vi "test2_2.vi"() -> ()   [LabVIEW 2010]
doc: "This example shows how to use the instrument's output voltage sweep mode. The actual voltage levels and actual current levels are returned as well as whether over current protection (OCP) has been tripped."
uses:
  <instrlib>/Agilent B2900 Series/Public/Configure/Measurement/Configure Measurement (Current).vi
  <instrlib>/Agilent B2900 Series/Public/Data/Low Level/Fetch Measurement (Multiple Points).vi
  <instrlib>/Agilent B2900 Series/Agilent B2900 Series.lvlib
panel:
  out "Resistance":dbl[](graph)
  out "Resistance":dbl[](array[numeric])
  out "Current vs Voltage":cluster{"Y":dbl[], "Y":dbl[]}[](graph)
  in  "Sweep Range Mode (2: Auto)":i32(ring)=2 items=["Best", "Fix", "Auto"]
  in  "Sweep Number of Steps (7)":i32=7
  in  "Sweep Stop (10 V)":dbl=10.0
  in  "Sweep Start (3 V)":dbl=3.0
  in  "Sweep Output Mode (0: Linear Single)":i32(ring) items=["Linear Single", "Linear Double", "Log Single", "Log Double"]
  out "Actual Voltage Levels (V)":dbl[](array[numeric])
  out "Actual Current Levels (A)":dbl[](array[numeric])
  out "OCP Tripped?":bool
  in  "Current NPLC (0.1)":dbl=0.1
  in  "Trigger Source (0: Auto-Internal)":i32(ring) items=["Auto-Internal", "Bus", "Timer", "INT1", "INT2", "LAN", "EXT1", "EXT2", "EXT3", "EXT4", "EXT5", "EXT6", "EXT7", "EXT8", "EXT9", "EXT10", "EXT11", "EXT12", "EXT13", "EXT14"]
  in  "Enable Output Protection(T: Enable)":bool=TRUE
  in  "Compliance Current (0.0001 A)":dbl=0.0001 format="%_3g"
  in  "Channel (0: Channel 1)":i32(ring) items=["Channel 1", "Channel 2"]
  in  "VISA resource name":refnum<visa-resource-name>
  # "(c) 2011-2013 National Instruments.  ALL RIGHTS RESERVED."
  # "Output Settings"
  # "Compliance Protection"
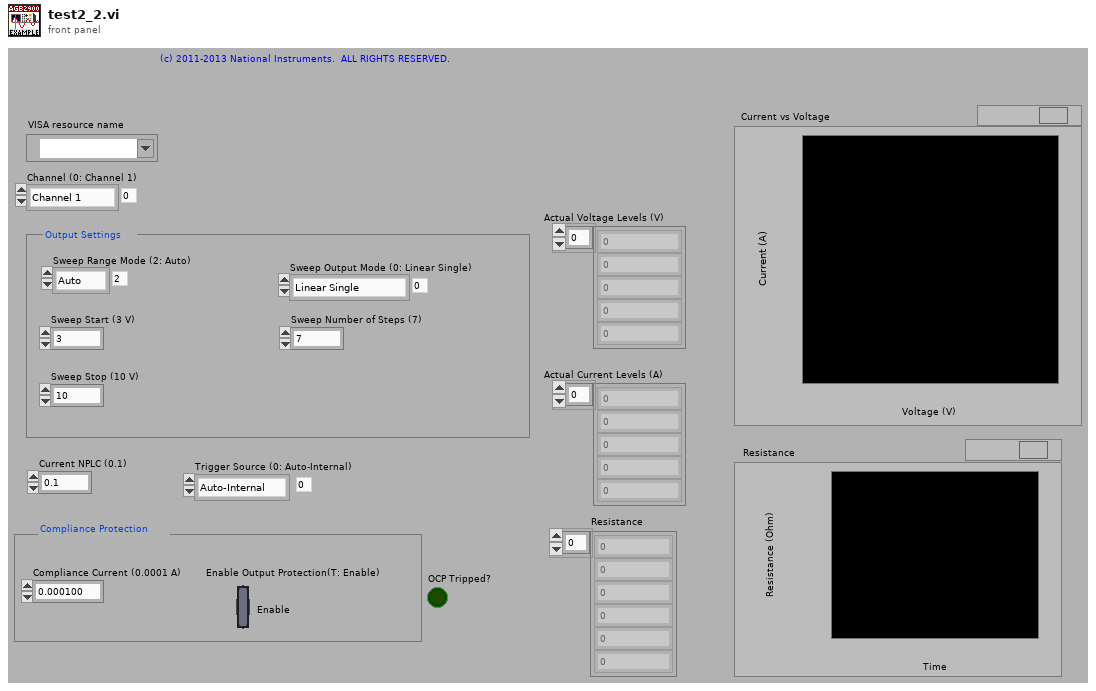
[diagram p1: front panel]
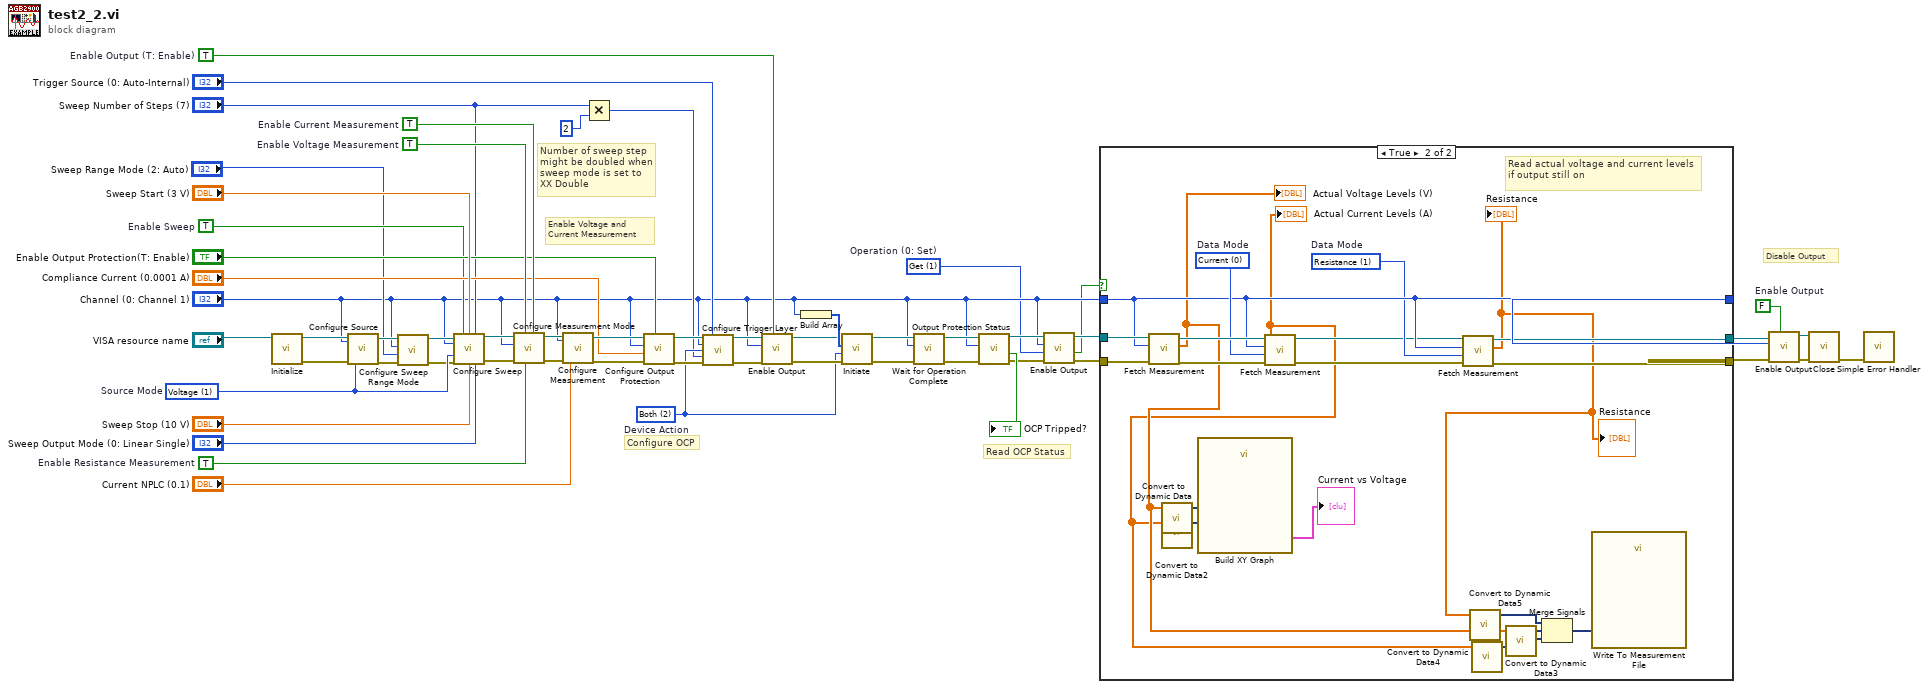
[diagram p0: block diagram]
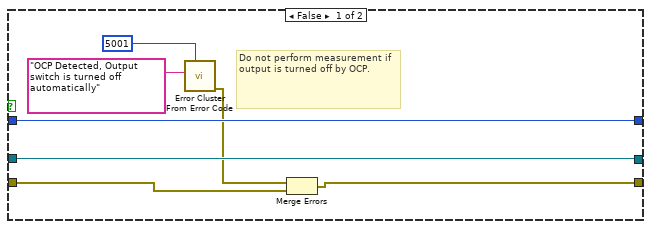
[diagram p2: hidden frame]
diagram:
  w3 = 1 items=["Set", "Get"]  # Operation (0: Set)
  w27 = TRUE  # Enable Current Measurement
  w28 = TRUE  # Enable Voltage Measurement
  w1 = FALSE  # Enable Output
  w26 = 2 items=["Acquire", "Transient", "Both"]  # Device Action
  w31 = TRUE  # Enable Resistance Measurement
  w21 = 1 items=["Current", "Voltage"]  # Source Mode
  w17 = TRUE  # Enable Sweep
  w55 = TRUE  # Enable Output (T: Enable)
  # "Number of sweep step \nmight be doubled when \nsweep mode is set to \nXX Double"
  # "Disable Output"
  # "Read OCP Status"
  # "Enable Voltage and \nCurrent Measurement"
  # "Configure OCP"
  n1 = call <instrlib>:"Initialize.vi"("VISA resource name"="VISA resource name") -> ("error out"=w29:errorcluster, "VISA resource name out"=w30:refnum<visa-resource-name>)  [unwired: 9 in]
  n2 = call <instrlib>:"Configure Source.vi"("VISA resource name"=w30, "Channel (0: Channel 1)"="Channel (0: Channel 1)", "error in (no error)"=w29, "Source Mode (1: Voltage)"=w21) -> ("VISA resource name out"=w15:refnum<visa-resource-name>, "error out"=w12:errorcluster)  [unwired: 14 in]
  n3 = call <instrlib>:"Configure Sweep Range Mode.vi"("error in (no error)"=w12, "Sweep Range Mode (2: Auto)"="Sweep Range Mode (2: Auto)", "Channel (0: Channel 1)"="Channel (0: Channel 1)", "VISA resource name"=w15) -> ("error out"=w13:errorcluster, "VISA resource name out"=w14:refnum<visa-resource-name>)  [unwired: 6 in]
  n4 = call <instrlib>:"Configure Sweep.vi"("VISA resource name"=w14, "Enable Sweep (F: Disable)"=w17, "Sweep Start (0)"="Sweep Start (3 V)", "Sweep Number of Steps (1)"="Sweep Number of Steps (7)", "Channel (0: Channel 1)"="Channel (0: Channel 1)", "Sweep Setting Mode (1: Voltage)"=w21, "error in (no error)"=w13, "Sweep Stop (0)"="Sweep Stop (10 V)", "Sweep Output Mode (0: Linear Single)"="Sweep Output Mode (0: Linear Single)") -> ("VISA resource name out"=w19:refnum<visa-resource-name>, "error out"=w18:errorcluster)  [unwired: 5 in]
  n5 = call <instrlib>:"Configure Measurement Mode.vi"("Enable Current Measurement (T: Enable)"=w27, "Enable Resistance Measurement (F: Disable)"=w31, "Enable Voltage Measurement (T: Enable)"=w28, "error in (no error)"=w18, "Channel (0: Channel 1)"="Channel (0: Channel 1)", "VISA resource name"=w19) -> ("error out"=w51:errorcluster, "VISA resource name out"=w52:refnum<visa-resource-name>)  [unwired: 4 in]
  n6 = call-poly <instrlib>:"Configure Measurement.vi"("VISA resource name"=w52, "Channel (0: Channel 1)"="Channel (0: Channel 1)", "error in (no error)"=w51, "Current NPLC (0.1)"="Current NPLC (0.1)") -> ("VISA resource name out"=w39:refnum<visa-resource-name>, "error out"=w38:errorcluster)  [unwired: 14 in]
  n7 = Multiply(x="Sweep Number of Steps (7)", y=2) -> (x*y=w24:i32)
  n8 = call <instrlib>:"Configure Output Protection.vi"("Enable Output Protection (T: Enable)"="Enable Output Protection(T: Enable)", "error in (no error)"=w38, "Compliance Current (0.0001 A)"="Compliance Current (0.0001 A)", "Channel (0: Channel 1)"="Channel (0: Channel 1)", "VISA resource name"=w39) -> ("error out"=w36:errorcluster, "VISA resource name out"=w37:refnum<visa-resource-name>)  [unwired: 5 in]
  n9 = call <instrlib>:"Configure Trigger Layer.vi"("VISA resource name"=w37, "Trigger Source (0: Auto-Internal)"="Trigger Source (0: Auto-Internal)", "Channel (0: Channel 1)"="Channel (0: Channel 1)", "Device Action (2: Both)"=w26, "Trigger Count (1)"=w24, "error in (no error)"=w36) -> ("VISA resource name out"=w35:refnum<visa-resource-name>, "error out"=w34:errorcluster)  [unwired: 8 in]
  n10 = call <instrlib>:"Enable Output.vi"("Enable Output (T: Enable)"=w55, "error in (no error)"=w34, "Channel (0: Channel 1)"="Channel (0: Channel 1)", "VISA resource name"=w35) -> ("error out"=w53:errorcluster, "VISA resource name out"=w54:refnum<visa-resource-name>)  [unwired: 5 in, 1 out]
  n11 = Build Array("Channel (0: Channel 1)") -> (w56:i32[])
  n12 = call <instrlib>:"Initiate.vi"("error in (no error)"=w53, "Device Action (2: Both)"=w26, "Channel List ({Channel1})"=w56, "VISA resource name"=w54) -> ("error out"=w32:errorcluster, "VISA resource name out"=w33:refnum<visa-resource-name>)  [unwired: 6 in]
  n13 = call <instrlib>:"Wait for Operation Complete.vi"("error in (no error)"=w32, "Channel (0: Channel 1)"="Channel (0: Channel 1)", "VISA resource name"=w33) -> ("error out"=w42:errorcluster, "VISA resource name out"=w43:refnum<visa-resource-name>)  [unwired: 7 in]
  n14 = call <instrlib>:"Output Protection Status.vi"("error in (no error)"=w42, "Channel (0: Channel 1)"="Channel (0: Channel 1)", "VISA resource name"=w43) -> ("error out"=w5:errorcluster, "OCP Tripped?"=→"OCP Tripped?":bool, "VISA resource name out"=w8:refnum<visa-resource-name>)  [unwired: 5 in, 1 out]
  n15 = call <instrlib>:"Enable Output.vi"("error in (no error)"=w5, "Operation (0: Set)"=w3, "Channel (0: Channel 1)"="Channel (0: Channel 1)", "VISA resource name"=w8) -> ("error out"=w7:errorcluster, "Output Enabled?"=w2:bool, "VISA resource name out"=w6:refnum<visa-resource-name>)  [unwired: 5 in]
  n16 = case shown="True" w2 {
    tunnel: w6 -> [w63 w85]
    tunnel: w7 -> [w58 w84]
    tunnel: [w60 w72] -> w41
    tunnel: [w63 w73] -> w40
    tunnel: "Channel (0: Channel 1)" -> [w64 w74]
    tunnel: [w64 w74] -> w10
    frame False {
      # "Do not perform measurement if output is turned off by OCP."
      n17 = call <vilib>:"Error Cluster From Error Code.vi"("error message (\"\")"="OCP Detected, Output switch is turned off automatically" ("error message (\"\")"), "error code (0)"=5001) -> ("error out"=w59:errorcluster)  [unwired: 7 in]
      n18 = Merge Errors(w59, w58) -> (w60:errorcluster)
    }
    frame True {
      w71 = 1 items=["Current", "Resistance", "Source Output Setting", "Status", "Time", "Voltage"]  # Data Mode
      w81 = 0 items=["Current", "Resistance", "Source Output Setting", "Status", "Time", "Voltage"]  # Data Mode
      # "Read actual voltage and current levels if output still on"
      n19 = call-poly <instrlib>:"Fetch Measurement.vi"("error in (no error)"=w84, "Channel (0: Channel 1)"=w74, "VISA resource name"=w85) -> ("error out"=w83:errorcluster, "Measurements"=w67:dbl[], "VISA resource name out"=w82:refnum<visa-resource-name>)  [unwired: 6 in]
      "Actual Voltage Levels (V)" <- w67
      n20 = call "Convert to Dynamic Data"("Array"=w67) -> ("Dynamic Data Type"=w79:dynamicdata)  [unwired: 3 in]
      n21 = call-poly <instrlib>:"Fetch Measurement.vi"("error in (no error)"=w83, "Data Mode (5: Voltage)"=w81, "Channel (0: Channel 1)"=w74, "VISA resource name"=w82) -> ("error out"=w70:errorcluster, "Measurements"=w66:dbl[], "VISA resource name out"=w69:refnum<visa-resource-name>)  [unwired: 5 in]
      "Actual Current Levels (A)" <- w66
      n22 = call "Convert to Dynamic Data2"("Array"=w66) -> ("Dynamic Data Type"=w78:dynamicdata)  [unwired: 3 in]
      n23 = call "Build XY Graph"("Y Input"=w78, "X Input"=w79) -> ("XY Graph"=→"Current vs Voltage":cluster{"Y":dbl[], "Y":dbl[]}[])  [unwired: 3 in, 6 out]
      n24 = call-poly <instrlib>:"Fetch Measurement.vi"("error in (no error)"=w70, "Data Mode (5: Voltage)"=w71, "Channel (0: Channel 1)"=w74, "VISA resource name"=w69) -> ("error out"=w72:errorcluster, "Measurements"=w65:dbl[], "VISA resource name out"=w73:refnum<visa-resource-name>)  [unwired: 5 in]
      "Resistance" <- w65
      "Resistance" <- w65
      n25 = call "Convert to Dynamic Data5"("Array"=w65) -> ("Dynamic Data Type"=w68:dynamicdata)  [unwired: 3 in]
      n26 = call "Convert to Dynamic Data4"("Array"=w66) -> ("Dynamic Data Type"=w76:dynamicdata)  [unwired: 3 in]
      n27 = call "Convert to Dynamic Data3"("Array"=w67) -> ("Dynamic Data Type"=w77:dynamicdata)  [unwired: 3 in]
      n28 = Merge Signals(w68, w77, w76) -> (w75:dynamicdata)
      n29 = call "Write To Measurement File"("Signals"=w75) -> ()  [unwired: 16 in, 3 out]
    }
  }
  n30 = call <instrlib>:"Enable Output.vi"("Enable Output (T: Enable)"=w1, "error in (no error)"=w41, "Channel (0: Channel 1)"=w10, "VISA resource name"=w40) -> ("error out"=w46:errorcluster, "VISA resource name out"=w45:refnum<visa-resource-name>)  [unwired: 5 in, 1 out]
  n31 = call <instrlib>:"Close.vi"("error in (no error)"=w46, "VISA resource name"=w45) -> ("error out"=w47:errorcluster)  [unwired: 9 in]
  n32 = call <vilib>:"Simple Error Handler.vi"("error in (no error)"=w47) -> ()  [unwired: 4 in, 5 out]
